vi "TF_Tacho2Velocity.vi"(1 "Tachometer Voltage [V]":dbl, 4 "Tachometer param":T1={"Offset [V]"=0.0, "Gain [deg/sV]"=130.0}) -> (0 "Tachometer Velocity [deg/s]":dbl)   [LabVIEW 2019]
uses:
  ModelSpecific/TypeDefTachometerParam.ctl
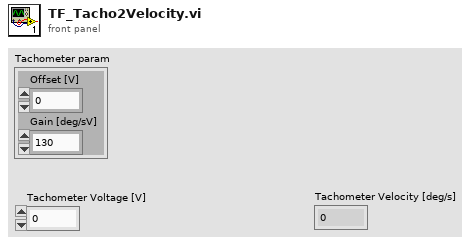
[diagram p1: front panel]
types:
  T1 = typedef "TypeDefTachometerParam.ctl" = cluster{"Offset [V]":dbl, "Gain [deg/sV]":dbl}
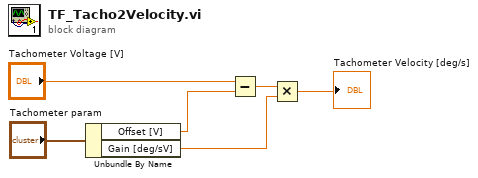
[diagram p0: block diagram]
diagram:
  n1 = Unbundle By Name("Tachometer param") -> ("Offset [V]"=w4:dbl, "Gain [deg/sV]"=w2:dbl)
  n2 = Subtract(x="Tachometer Voltage [V]", y=w4) -> (x-y=w3:dbl)
  n3 = Multiply(x=w3, y=w2) -> (x*y=→"Tachometer Velocity [deg/s]":dbl)
